vi "Arm Control.vi"(6 "bottom":bool, 7 "top":bool, 8 "Channels":string[](array[string]), 10 "Motor":dbl, 11 "Enum":T1) -> ()   [LabVIEW 2014]
uses:
  SRE Enum.ctl
  Text Variable VIs/Read Number Variable.vi
  <vilib>/Rock Robotics/WPI/MotorControl/WPI_MotorControlOpen Talon.vi
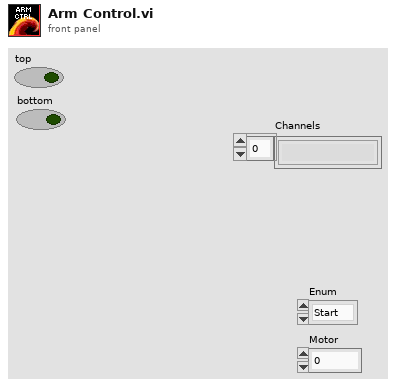
[diagram p1: front panel]
types:
  T1 = typedef "SRE Enum.ctl" = enum16{"Start", "Run", "End"}
  T2 = typedef "WPI_MotorControlDeviceRef.ctl" = cluster{"DeviceStatus":errorcluster, "Type":T3, "PWM":cluster{"Controller":T4, "PWM Channel":T5, "DeadBand":T6}, "CAN":cluster{"Device Number":u8, "Control Mode":T7, "Semaphore":T8, "Max Vout":dbl, "TalonSRX Control Mode":T9}, "Invert":bool, "TransformRef":T10, "InvTransformRef":T10}
  T3 = typedef "WPI_MotorControlType.ctl" = enum16{"PWM", "CAN", "CANTalonSRX"}
  T4 = typedef "FPGA_TypedefDigitalModule.ctl" = enum16{"Controller 1"}
  T5 = typedef "FPGA_DIOPWMChannel.ctl" = enum8{"PWM 0", "PWM 1", "PWM 2", "PWM 3", "PWM 4", "PWM 5", "PWM 6", "PWM 7", "PWM 8", "PWM 9", "PWM MXP 0", "PWM MXP 1", "PWM MXP 2", "PWM MXP 3", "PWM MXP 4", "PWM MXP 5", "PWM MXP 6", "PWM MXP 7", "PWM MXP 8", "PWM MXP 9", "Invalid"}
  T6 = typedef "WPI_PWMDeadband.ctl" = cluster{"Name":string, "maxPositivePwm":i32, "minPositivePwm":i32, "centerPwm":i32, "maxNegativePwm":i32, "minNegativePwm":i32, "angularRange":u16}
  T7 = typedef "WPI_CANJaguar_ControlMode.ctl" = enum8{"Percent VBus", "Current", "Speed", "Position", "Voltage"}
  T8 = typedef "Semaphore RefNum" = refnum<k1>
  T9 = typedef "WPI_CANTalonSRX_APIControlMode.ctl" = enum8{"Percent VBus", "Speed", "Position", "Slave", "Unchanged / Invalid"}
  T10 = typedef "WPI_PWMTransform_ConPane.ctl" = refnum<vi>
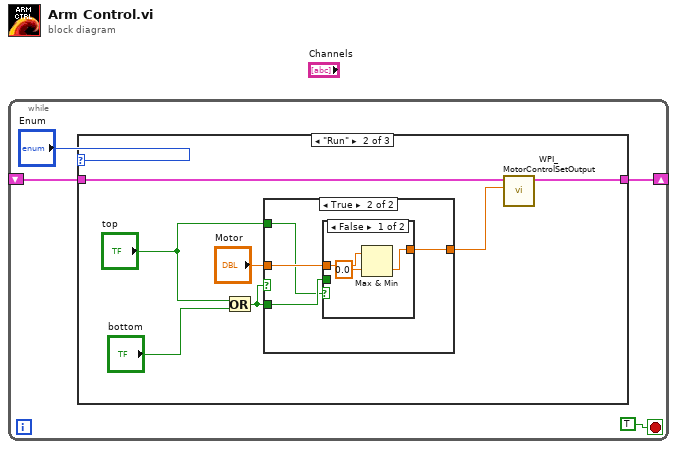
[diagram p0: block diagram]
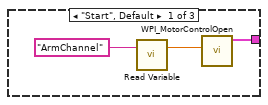
[diagram p2: hidden frame]
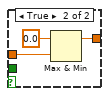
[diagram p4: hidden frame]
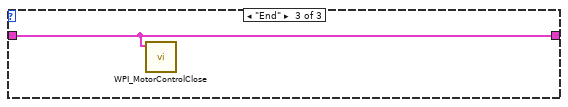
[diagram p5: hidden frame]
diagram:
  n1 = while {
    shift-right: [w4] -> _
    shift-left: _ -> [w3]
    stop <- TRUE stop-if-true
    n2 = case shown="\"Run\"" "Enum" {
      tunnel: [w5 w12 w26] -> w4
      tunnel: w3 -> [_ w11 w26]
      frame "Start", Default {
        n3 = call-poly "Read Variable.vi"("Name"="ArmChannel") -> ("number"=w6:dbl)  [unwired: 1 in, 1 out]
        n4 = call-poly <vilib>:"WPI_MotorControlOpen.vi"("PWM Channel"=w6) -> ("MotorControlDeviceRef"=w5:T2)  [unwired: 9 in, 1 out]
      }
      frame "Run" {
        n5 = Or(x="top", y="bottom") -> (x .or. y?=w14:bool)
        n6 = case shown="True" w14 {
          tunnel: w14 -> [_ w19]
          tunnel: "Motor" -> [w15 w18]
          tunnel: [w15 w17] -> w13
          tunnel: "top" -> [_ w16]
          frame False {
          }
          frame True {
            n7 = case shown="False" w16 {
              tunnel: w19 -> [_ _]
              tunnel: w18 -> [w21 w25]
              tunnel: [w22 w23] -> w17
              frame False {
                n8 = Max & Min(x=w21, y=0.0) -> (min(x,y)=w22:dbl)  [unwired: 1 out]
              }
              frame True {
                n9 = Max & Min(x=0.0, y=w25) -> (max(x,y)=w23:dbl)  [unwired: 1 out]
              }
            }
          }
        }
        n10 = call <vilib>:"WPI_MotorControlSetOutput.vi"("Output"=w13, "MotorControlDevRef"=w11) -> ("MotorControlDevRef"=w12:T2)  [unwired: 7 in, 2 out]
      }
      frame "End" {
        n11 = call <vilib>:"WPI_MotorControlClose.vi"("MotorControlDevRef"=w26) -> ()  [unwired: 10 in, 1 out]
      }
    }
  }
